vi "GT Arc XYZWN.vi"(0 "cardNum":i16, 1 "crd":i16, 2 "x":i32, 3 "y":i32, 4 "z":i32, 5 "interX":dbl, 6 "interY":dbl, 7 "error in (no error)":errorcluster caption="错误输入（无错误）", 8 "interZ":dbl, 9 "synVel":dbl, 10 "synAcc":dbl, 11 "velEnd":dbl, 12 "segNum":i32, 13 "fifo":i16) -> (20 "function return":i16, 27 "error out":errorcluster caption="错误输出")   [LabVIEW 2020, in "gts.lvlib"]
doc: "GT_API GT_ArcXYZWN(short cardNum,short crd,long x,long y,long z,double interX,double interY,double interZ,double synVel,double synAcc,double velEnd=0,long segNum=0,short fifo=0);"
uses:
  gts.lvlib
  dll/32bit/multi_card/gts.dll
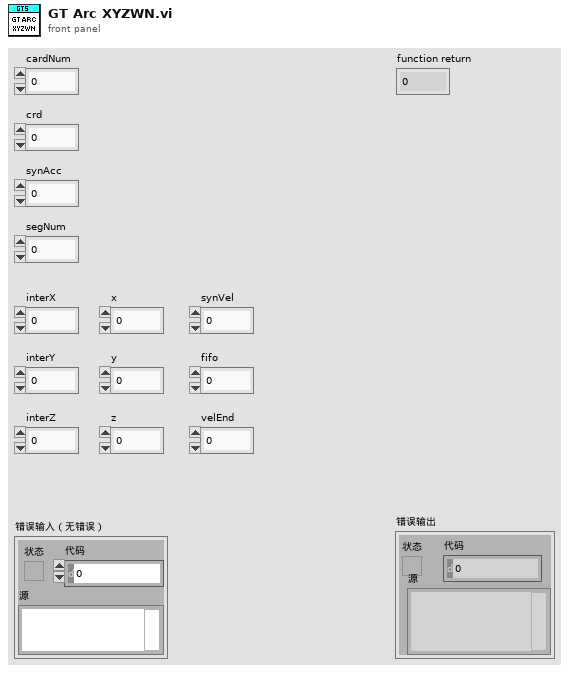
[diagram p1: front panel]
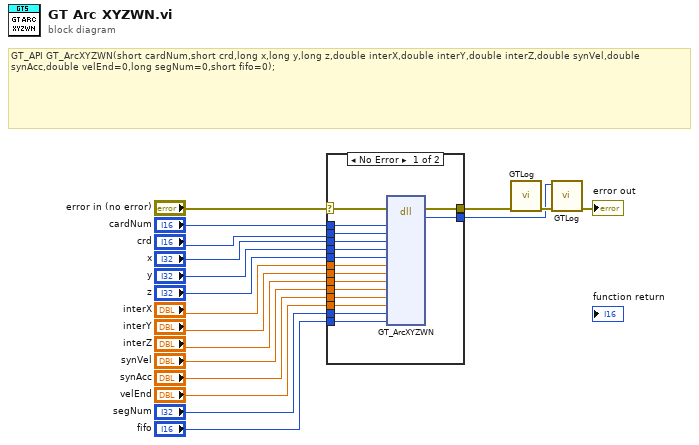
[diagram p0: block diagram]
diagram:
  # "GT_API GT_ArcXYZWN(short cardNum,short crd,long x,long y,long z,double interX,double interY,double interZ,double synVel,double synAcc,double velEnd=0,long segNum=0,short fifo=0);"
  n1 = case shown="No Error" "error in (no error)" {
    selector: "error in (no error)" -> [w20 w35]
    tunnel: [w34 _] -> w1
    tunnel: "cardNum" -> [w33 _]
    tunnel: "crd" -> [w32 _]
    tunnel: "x" -> [w31 _]
    tunnel: "y" -> [w30 _]
    tunnel: "z" -> [w29 _]
    tunnel: "interX" -> [w28 _]
    tunnel: "interY" -> [w27 _]
    tunnel: "interZ" -> [w26 _]
    tunnel: "synVel" -> [w25 _]
    tunnel: "synAcc" -> [w24 _]
    tunnel: "velEnd" -> [w23 _]
    tunnel: "segNum" -> [w22 _]
    tunnel: "fifo" -> [w21 _]
    tunnel: [w19 w35] -> w4
    frame No Error {
      n2 = dll-call lib="C:/1228/dll/32bit/multi_card/gts.*" fn="GT_ArcXYZWN"(error in=w20, "cardNum"=w33, "crd"=w32, "x"=w31, "y"=w30, "z"=w29, "interX"=w28, "interY"=w27, "interZ"=w26, "synVel"=w25, "synAcc"=w24, "velEnd"=w23, "segNum"=w22, "fifo"=w21) -> (error out=w19:errorcluster, w34:i16)  [unwired: 15 in, 1 out]
    }
    frame Error {
    }
  }
  n3 = call "GTLog.vi"("error in (no error)"=w4) -> ("error out"=w3:errorcluster)  [unwired: 10 in]
  n4 = call "GTLog.vi"("error in (no error)"=w3, "Numeric"=w1) -> ("error out"=→"error out":errorcluster)  [unwired: 9 in]
